vi "hamamatsuRunSingleVolumes.vi"() -> ()   [LabVIEW 2017]
uses:
  globalUtilities.vi
  globalDevices.vi
panel:
  out "Waveform Chart":i32[](graph)
  out "frameAvailable":i32[](array[numeric])
  out "Data":u16[][][](array[numeric])
  in  "get volume":bool
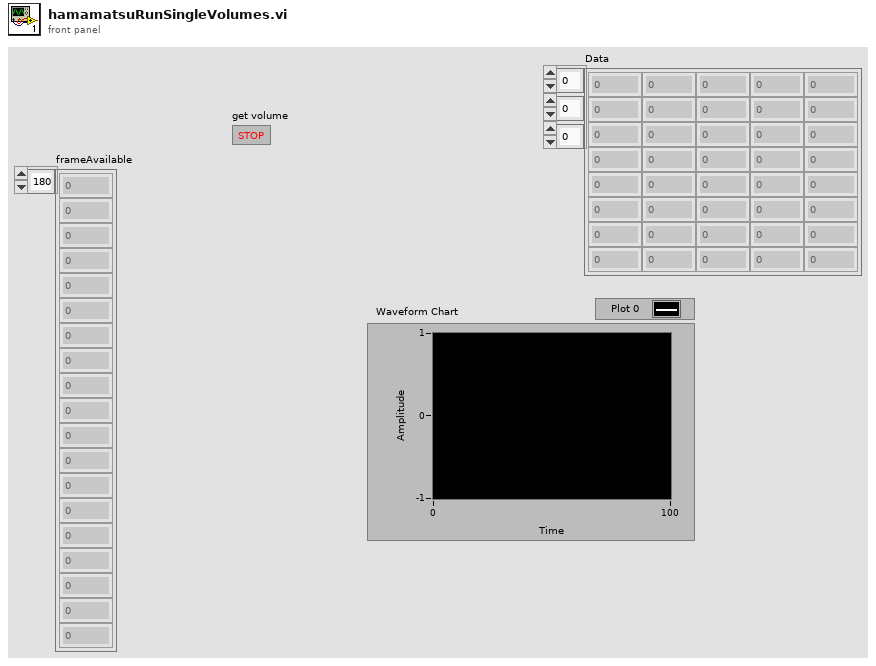
[diagram p1: front panel]
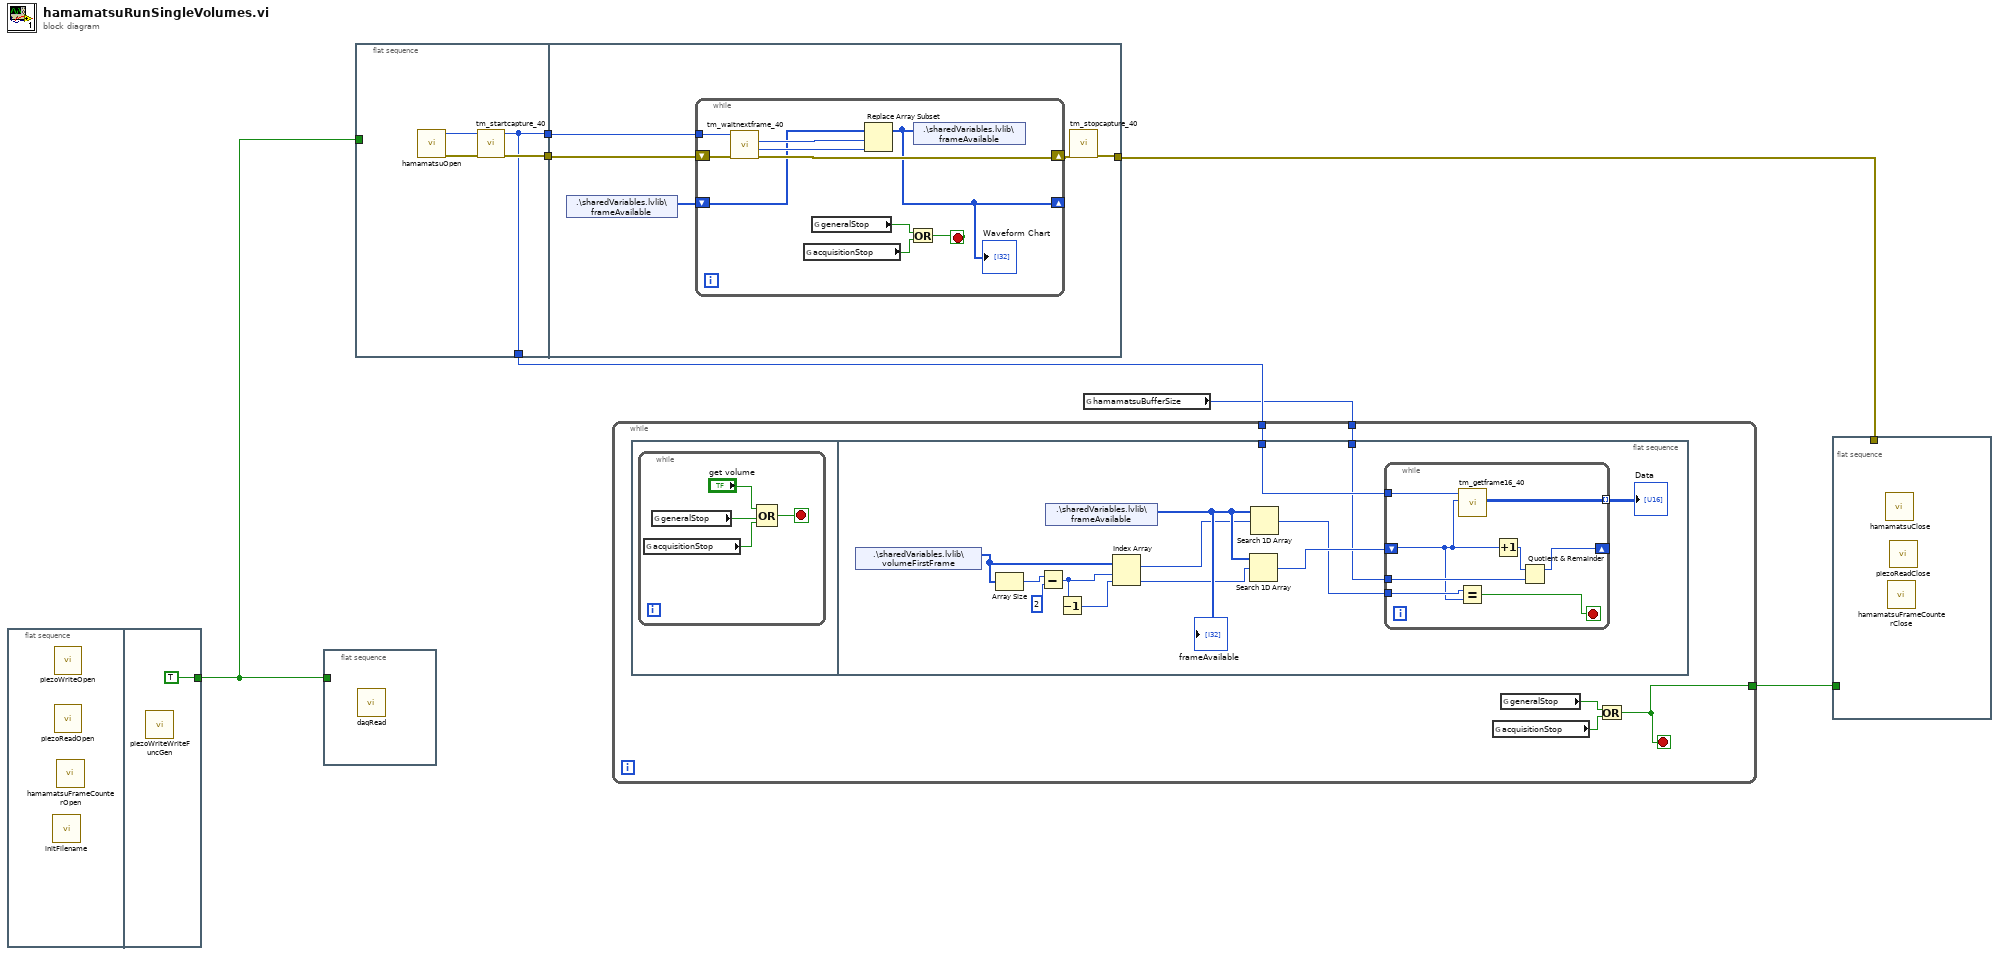
[diagram p0: block diagram]
diagram:
  n1 = flat-sequence {
    tunnel: [TRUE] -> w5
    frame #0 {
      n2 = call "initFilename.vi"() -> ()  [unwired: 2 in, 1 out]
      n3 = call "piezoWriteOpen.vi"() -> ()  [unwired: 2 in]
      n4 = call "piezoReadOpen.vi"() -> ()  [unwired: 6 in]
      n5 = call "hamamatsuFrameCounterOpen.vi"() -> ()  [unwired: 12 in]
    }
    frame #1 {
      n6 = call "piezoWriteWriteFuncGen.vi"() -> ()  [unwired: 12 in]
    }
  }
  n7 = flat-sequence {
    tunnel: w5 -> [_]
    frame #0 {
      n8 = call "daqRead.vi"() -> ()  [unwired: 3 in]
    }
  }
  n9 = flat-sequence {
    tunnel: [w10] -> w7
    tunnel: [w9] -> w6
    tunnel: w5 -> [_]
    tunnel: [w9] -> w4
    tunnel: w7 -> [w16]
    tunnel: w6 -> [w17]
    tunnel: [w14] -> w2
    frame #0 {
      n10 = call "hamamatsuOpen.vi"() -> ("error out"=w12:errorcluster, "Handle out"=w11:u32)  [unwired: 2 out]
      n11 = call <userlib>:"tm_startcapture_40.vi"("error in (no error)"=w12, "Handle in"=w11) -> ("error out"=w10:errorcluster, "Handle out"=w9:u32)  [unwired: 8 in]
    }
    frame #1 {
      n12 = shared-variable ".\\sharedVariables.lvlib\\frameAvailable"() -> (w13:i32[])  [unwired: 1 in, 1 out]
      n13 = while {
        tunnel: w17 -> [w27]
        shift-right: [w22] -> w15
        shift-left: w16 -> [w26]
        shift-right: [w18] -> _
        shift-left: w13 -> [w19]
        stop <- w23 stop-if-true
        n14 = call <userlib>:"tm_waitnextframe_40.vi"("error in (no error)"=w26, "Handle in"=w27) -> ("error out"=w22:errorcluster, "Frame Count"=w20:i32, "Frame Index"=w21:i32)  [unwired: 6 in, 1 out]
        n15 = global read "globalUtilities.vi" "acquisitionStop"() -> (w24:bool)
        n16 = global read "globalUtilities.vi" "generalStop"() -> (w25:bool)
        n17 = Replace Array Subset(array=w19, new element=w20, index=w21) -> (w18:i32[])
        "Waveform Chart" <- w18
        n18 = Or(x=w25, y=w24) -> (x .or. y?=w23:bool)
        n19 = shared-variable ".\\sharedVariables.lvlib\\frameAvailable"(w18) -> ()  [unwired: 1 in, 1 out]
      }
      n20 = call <userlib>:"tm_stopcapture_40.vi"("error in (no error)"=w15) -> ("error out"=w14:errorcluster)  [unwired: 9 in, 1 out]
    }
  }
  n21 = global read "globalDevices.vi" "hamamatsuBufferSize"() -> (w1:i32)
  n22 = while {
    tunnel: w4 -> [w30]
    tunnel: [w29] -> w3
    tunnel: w1 -> [w28]
    stop <- w29 stop-if-true
    n23 = flat-sequence {
      tunnel: w30 -> [w47]
      tunnel: w28 -> [w38]
      frame #0 {
        n24 = while {
          stop <- w33 stop-if-true
          n25 = global read "globalUtilities.vi" "acquisitionStop"() -> (w34:bool)
          n26 = global read "globalUtilities.vi" "generalStop"() -> (w35:bool)
          n27 = Compound Arithmetic op=OR("get volume", w35, w34) -> (w33:bool)
        }
      }
      frame #1 {
        n28 = shared-variable ".\\sharedVariables.lvlib\\volumeFirstFrame"() -> (w46:u32[])  [unwired: 1 in, 1 out]
        n29 = Array Size(array=w46) -> (size(s)=w40:i32)
        n30 = Subtract(x=w40, y=2) -> (x-y=w45:i32)
        n31 = shared-variable ".\\sharedVariables.lvlib\\frameAvailable"() -> (w49:i32[])  [unwired: 1 in, 1 out]
        "frameAvailable" <- w49
        n32 = Decrement(x=w45) -> (x-1=w44:i32)
        n33 = Index Array(array=w46, index #1=w45, index #2=w44) -> (element #1=w43:u32, element #2=w42:u32)
        n34 = Search 1D Array(1D array=w49, element=w42) -> (index of element=w48:i32)  [unwired: 1 in]
        n35 = Search 1D Array(1D array=w49, element=w43) -> (index of element=w37:i32)  [unwired: 1 in]
        n36 = while {
          tunnel: w47 -> [w57]
          shift-right: [w53] -> _
          shift-left: w48 -> [w51]
          tunnel: [w56] -> w41 mode=indexing
          tunnel: w38 -> [w55]
          tunnel: w37 -> [w52]
          stop <- w50 stop-if-true
          n37 = call <userlib>:"tm_getframe16_40.vi"("Frame Index"=w51, "Handle in"=w57) -> ("Data"=w56:u16[][])  [unwired: 6 in, 3 out]
          n38 = Equal?(x=w52, y=w51) -> (x = y?=w50:bool)
          n39 = Increment(x=w51) -> (x+1=w54:i32)
          n40 = Quotient & Remainder(x=w54, y=w55) -> (x-y*floor(x/y)=w53:i32)  [unwired: 1 out]
        }
        "Data" <- w41
      }
    }
    n41 = global read "globalUtilities.vi" "acquisitionStop"() -> (w32:bool)
    n42 = global read "globalUtilities.vi" "generalStop"() -> (w31:bool)
    n43 = Or(x=w31, y=w32) -> (x .or. y?=w29:bool)
  }
  n44 = flat-sequence {
    tunnel: w3 -> [_]
    tunnel: w2 -> [_]
    frame #0 {
      n45 = call "hamamatsuClose.vi"() -> ()  [unwired: 1 out]
      n46 = call "hamamatsuFrameCounterClose.vi"() -> ()  [unwired: 12 in]
      n47 = call "piezoReadClose.vi"() -> ()  [unwired: 1 in]
    }
  }
